vi "Ensaio_Jiga.vi"() -> ()   [LabVIEW 2025]
uses:
  Enum_Estados_Ensaio.ctl
  <vilib>/DAQmx/write.llb/DAQmx Write (Digital Bool 1Line 1Point).vi
  <vilib>/DAQmx/write.llb/DAQmx Write (Digital 1D Bool 1Chan 1Samp).vi
  <vilib>/Plasmionique/MB Master/MB_Master_Serial/MB_Master_Serial.lvclass
  C:/Program Files/National Instruments/LabVIEW 2025/vi.lib/Plasmionique/MB Master/MB_Master/MB_Master.lvclass
  <vilib>/DAQmx/create/channels.llb/DAQmx Create Channel (DO-Digital Output).vi
  <vilib>/DAQmx/miscellaneous.llb/DAQmx Fill In Error Info.vi
  <vilib>/Utility/file.llb/Write Delimited Spreadsheet (DBL).vi
  <vilib>/addons/control/pid/pid.llb/PID Gain Schedule (DBL).vi
  <vilib>/addons/control/pid/pid.llb/PID Advanced (DBL).vi
  <vilib>/Utility/file.llb/Write Delimited Spreadsheet (string).vi
  <instrlib>/Yokogawa PZ4000/Yokogawa PZ4000.lvlib
  <instrlib>/Yokogawa WT200 Series/Yokogawa WT200 Series.lvlib
  <vilib>/addons/control/pid/NI_PID_pid.lvlib
panel:
  out "Chart_velo":cluster{"V(A)":dbl, "V(B)":dbl}(graph)
  out "error out":errorcluster
  out "Registers":u16[](array[numeric])
  in  "Manual?":bool=TRUE
  in  "Medição contínua?":bool
  in  "Tempo de Integração":dbl=5.0
  in  "Realiza medição WT230":bool
  out "Tensão de Saída":dbl
  out "Corrente de Saída":dbl
  in  "Limite Tensao":dbl=24.0 min=0.0 max=36.0 step=0.5
  in  "Limite Corrente":dbl min=0.0 max=0.2 step=0.01
  in  "Para Freio":bool
  in  "Seta Carga":bool
  in  "Liga Fonte":bool
  in  "Iniciar Ensaio":bool
  in  "Finalizar Sessão":bool
  in  "ABORTAR":bool
  in  "?":T1(tab)
  out "Ensaio Rodando":bool
  in  "N_Resistores":string="1000"
  in  "Qtd. Braços Ativos":dbl min=0.0 max=7.0 step=1.0
  in  "Tempo de Pré-Carga (s)":dbl=90.0
  in  "Tempo de Acionamento do Motor (s)":dbl=14.0
  in  "Salvar Ensaio":path
  in  "VISA Resource":refnum<visa-resource-name>="COM3"
  in  "velocidade":u16
  in  "Serial Config":T2={"baud rate (bps)"=9600, "stop bits"=10, "parity"=2, "flow control"=0, "timeout"=2000, "retries"=3} {"stop bits" items=["1.0"=10, "1.5"=15, "2.0"=20]; "flow control" items=["None", "XON/XOFF", "RTS/CTS", "XON/XOFF & RTS/CTS", "DTR/DSR", "XON/XOFF & DTR/DSR"]; "parity" items=["None", "Odd", "Even", "Mark", "Space"]}
  in  "habilitar":u16=256
  out "Ganho atual do PI MI":T3={"proportional gain (Kc)"=100.0, "integral time (Ti, min)"=0.0, "derivative time (Td, min)"=0.0} {"derivative time (Td, min)" format="%.3f"; "integral time (Ti, min)" format="%.3f"; "proportional gain (Kc)" format="%.5f"}
  in  "SP_Power":i32
  out "Tempo Decorrido Acionamento Motor":dbl
  in  "Resistor 2 068":bool caption="4º Resistor 2 068"
  in  "Resistor 2 047":bool caption="3º Resistor 2 047"
  in  "Resistor 1  047":bool caption="2º Resistor 1  047"
  in  "Resistor 1 MOSFET":bool caption="1º Resistor 1 MOSFET"
  in  "PARAR WHILE":bool
  out "Estado Atual":T4
  out "V Cluster":cluster{"V(A)":dbl, "V(B)":dbl, "V(E)":dbl}
  out "I Cluster":cluster{"V(A)":dbl, "V(B)":dbl, "V(E)":dbl}
  out "P Cluster":T5
  out "PV_PowerControl":dbl
  in  "Ganhos PI do Gain Scheduling":T6(array[cluster])=[{"PID Parameters"={"Kc"=0.00026, "  Ti"=0.027, " Td"=0.0}, "Max PV"=490.0}, {"PID Parameters"={"Kc"=0.00027, "  Ti"=0.037, " Td"=0.0}, "Max PV"=690.0}, {"PID Parameters"={"Kc"=0.00019, "  Ti"=0.024, " Td"=0.0}, "Max PV"=900.0}] {"Max PV" format="%#.2f"; "PID Parameters"."Td" format="%#.3g"; "PID Parameters"."Ti" format="%#.3g"; "PID Parameters"."Kc" format="%#.5f"}
  in  "Ts Controle":dbl=0.1
  out "MV_MI":dbl=5.583364480052211
  out "Grafico_VelocidadeMotor":u16[](graph) caption="Velocidade do Motor"
  in  "Logfile_Watt":string="medsWatt"
  in  "Logfile_Freio":string="medsFreio"
  out "t":dbl
  in  "Logfile_ETMI":string="medsETMI"
  out "Corrente":dbl[][](graph)
  out "Tensão":dbl[][](graph)
  out "Graf_MV_MI":dbl(graph)
  out "Grafico_PowerControl":cluster{"PV_PowerControl":dbl, "SP_Power":i32}(graph)
  in  "Iniciar Acionamento":bool
  # "Aquisição WT230"
  # "CONTROLES DO ENSAIO"
  # "FREIO DE HISTERESE"
  # "Motor"
  # "Atenção: Antes de todo ensaio configurar o arquivo de saída para o padrão - Ensaio_{QtdBracos}bracos_RSE{ValorRSE}_SemCarga_{DataHora}.csv"
  # "Exemplo: 0Bracos_R1000_80W_2026-09-17_14_00.csv"
  # "BRAÇOS DE RESISTORES"
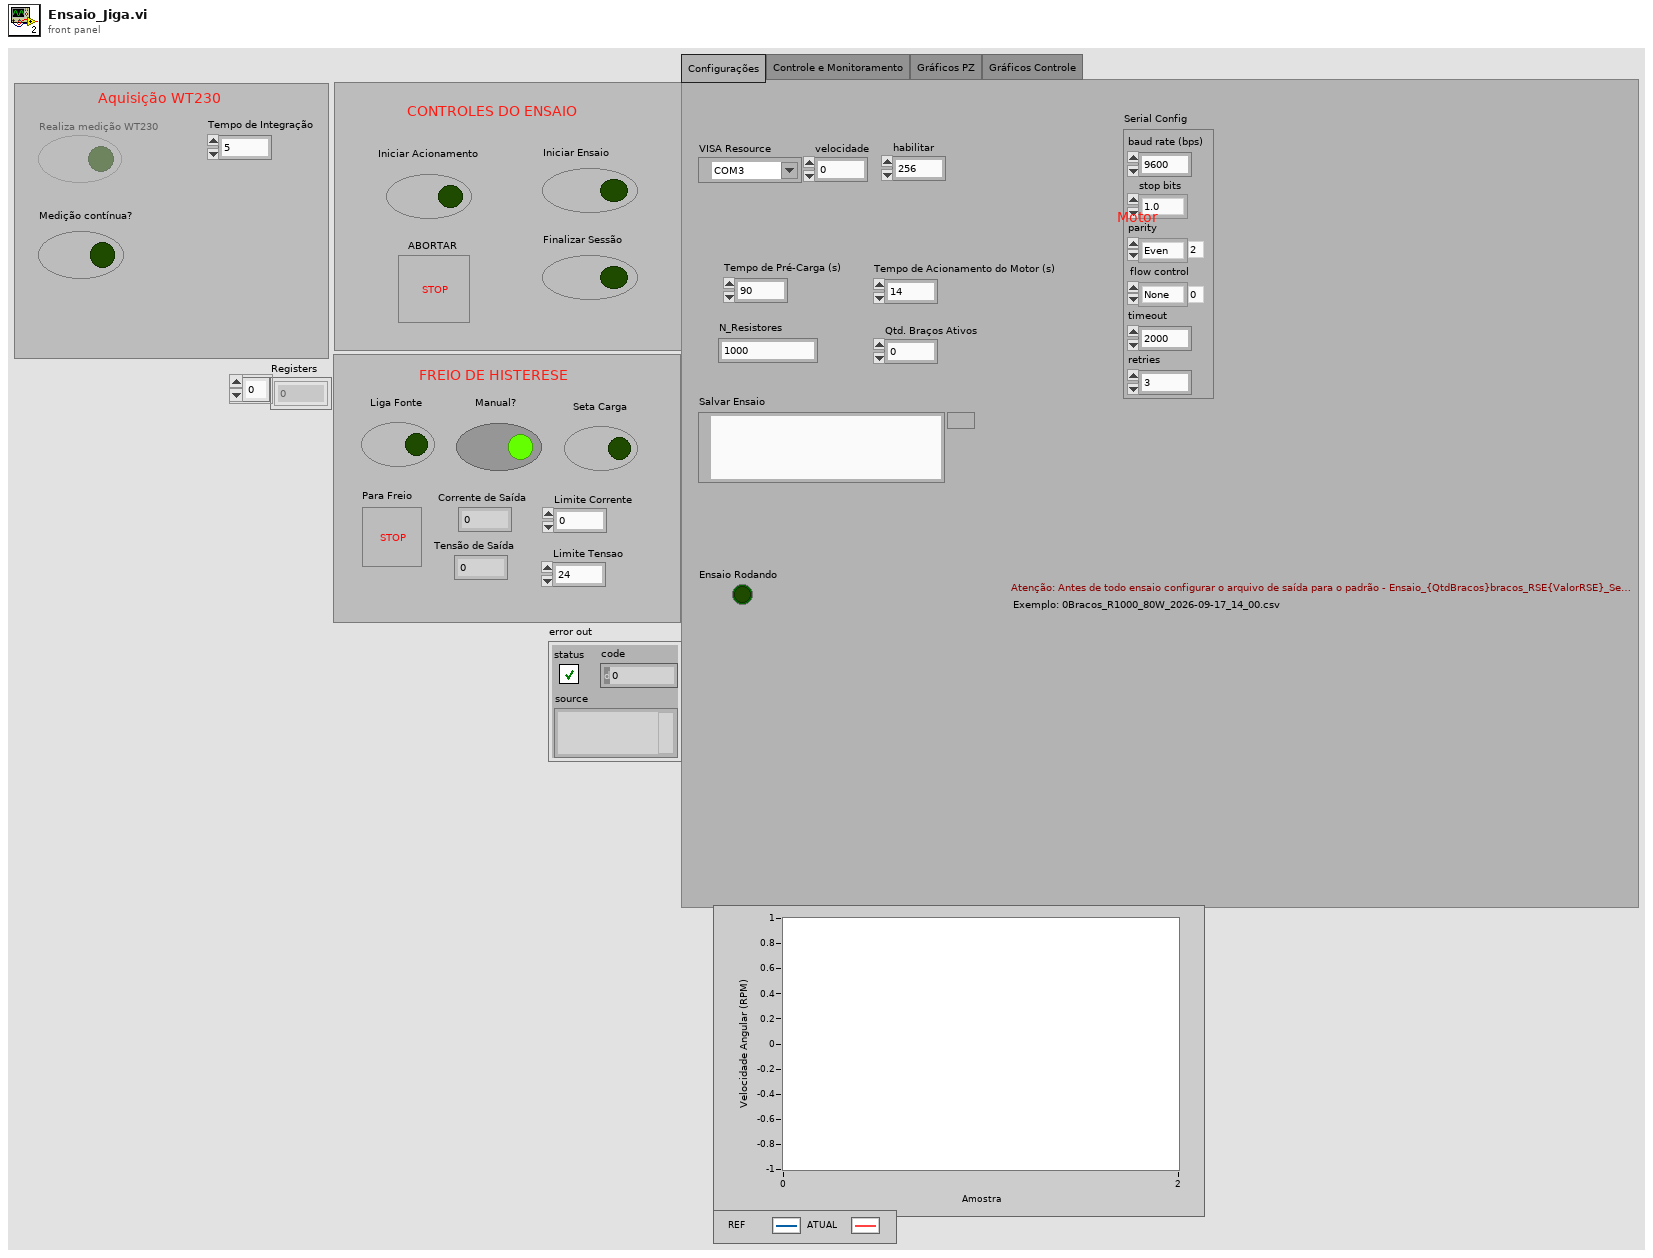
[diagram p1: front panel]
types:
  T1 = enum32{"Configurações", "Controle e Monitoramento", "Gráficos PZ", "Gráficos Controle"}
  T2 = cluster{"baud rate (bps)":u32, "stop bits":u16, "parity":u16, "flow control":u16, "timeout":u32, "retries":i32}
  T3 = cluster{"proportional gain (Kc)":dbl, "integral time (Ti, min)":dbl, "derivative time (Td, min)":dbl}
  T4 = typedef "Enum_Estados_Ensaio.ctl" = enum16{"Idle", "Pre_Carga", "Aguarda_PreCarga", "Ativa_Bracos", "Delay_PosBracos", "Desativa_PreCarga", "Aciona_Motor", "Aguarda_Motor", "Motor_Rodando", "Ensaio", "Para_Motor", "Emergencia\n"}
  T5 = cluster{"output":dbl, "output":dbl, "output":dbl, "PL(A)":dbl, "PL(B)":dbl, "PL(T)":dbl, "output":dbl, "PL(E)":dbl}
  T6 = cluster{"PID Parameters":cluster{"Kc":dbl, "  Ti":dbl, " Td":dbl}, "Max PV":dbl}[]
  T7 = enum8{"Enabled", "Disabled", "Disabled and Grayed Out"}
  T8 = cluster{"V(A)":dbl, "I(A)":dbl, "V(B)":dbl, "I(B)":dbl, "PC(A)":dbl, "PC(B)":dbl, "PC(T)":dbl, "PL(T)":dbl, "PL(B)":dbl, "PL(A)":dbl, "V(E)":dbl, "PL(E)":dbl, "PC(E)":dbl, "I(E)":dbl, "t":dbl}
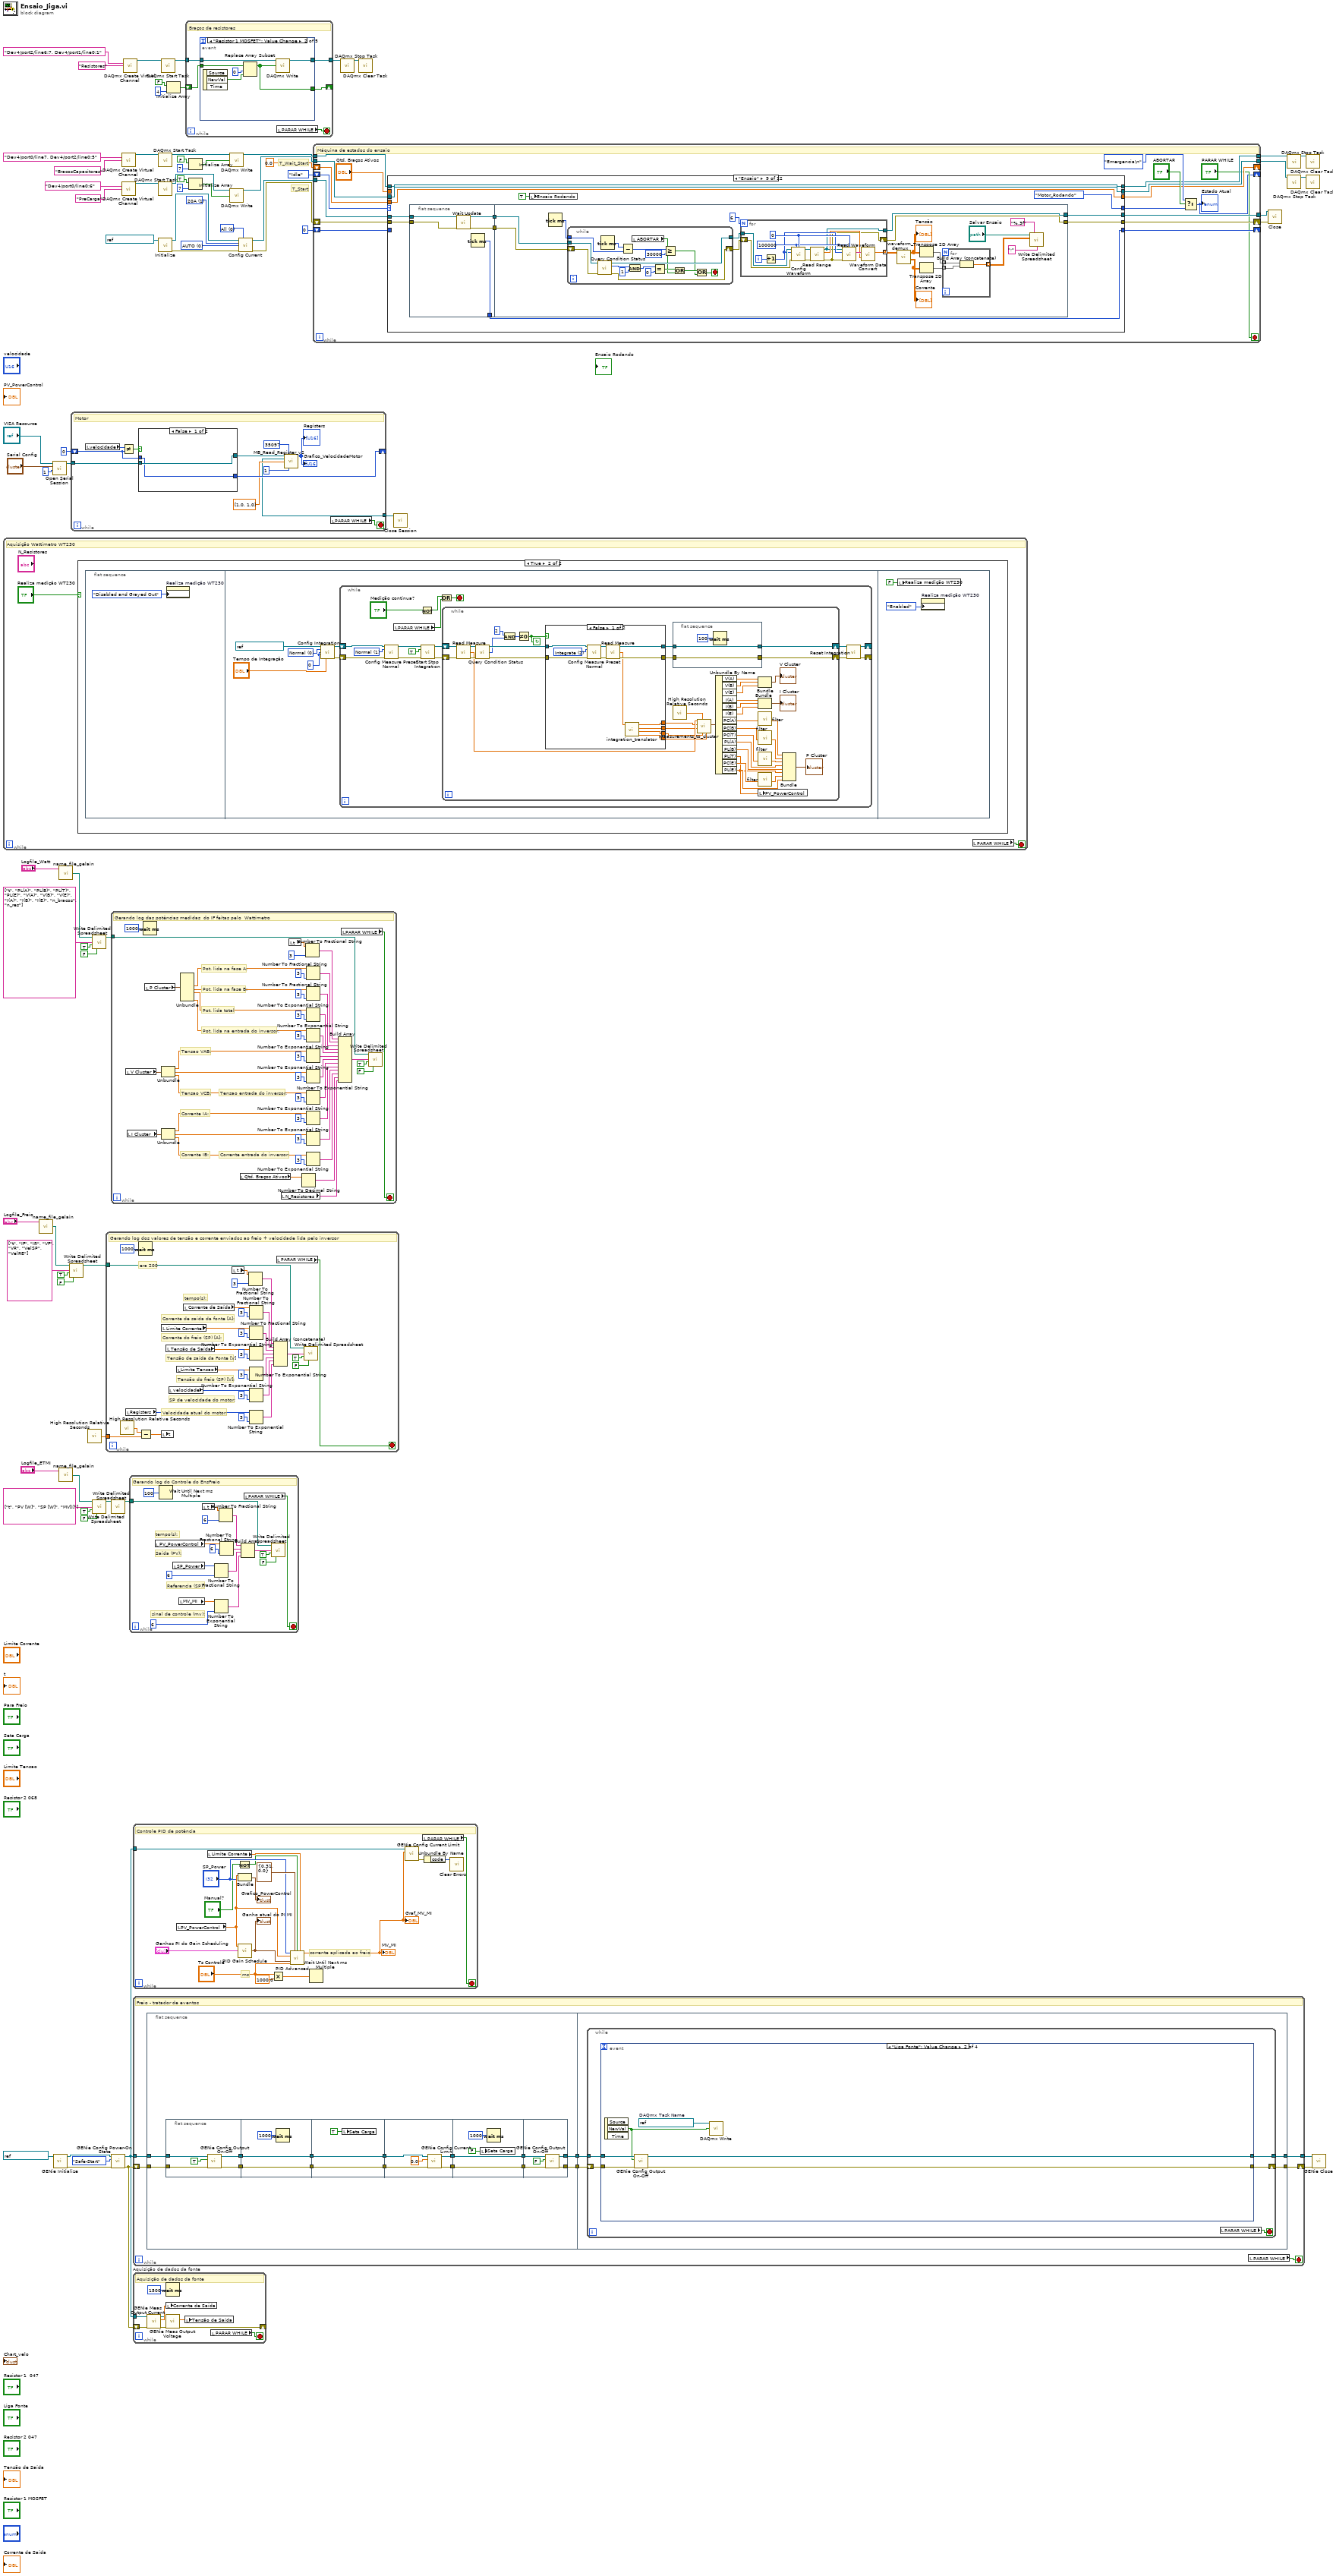
[diagram p0: block diagram]
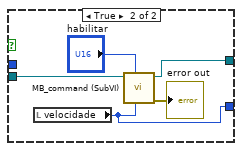
[diagram p2: hidden frame]
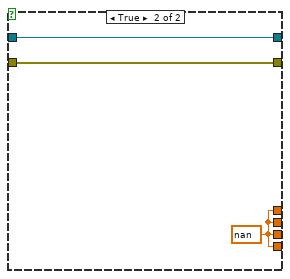
[diagram p4: hidden frame]
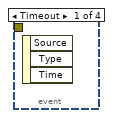
[diagram p5: hidden frame]
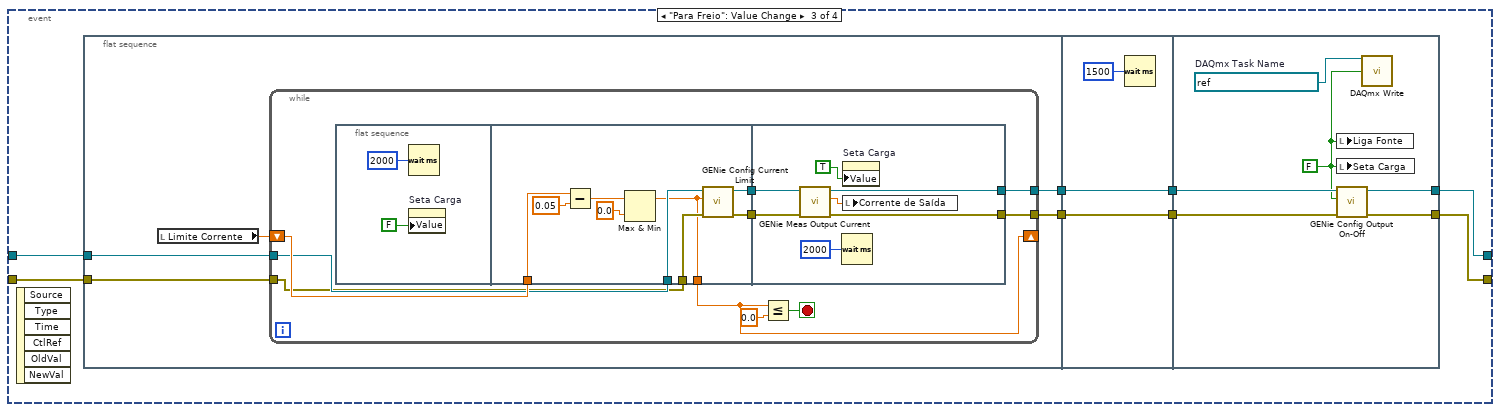
[diagram p6: hidden frame]
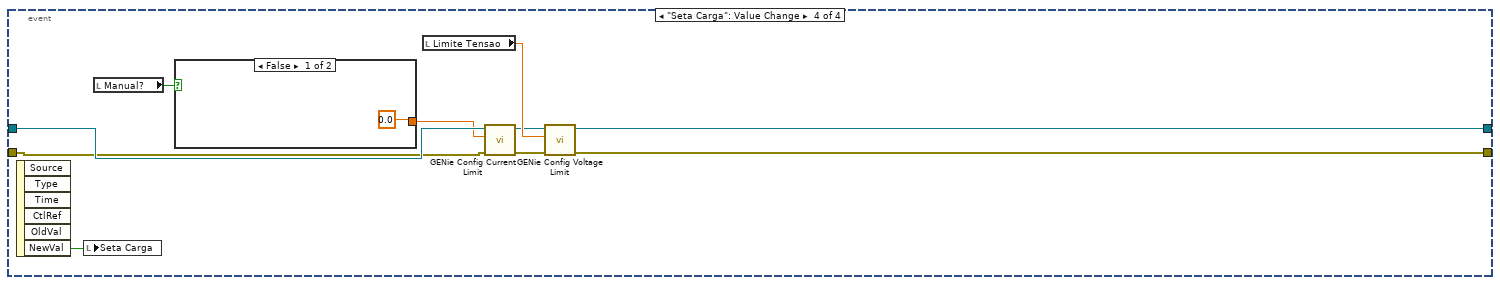
[diagram p7: hidden frame]
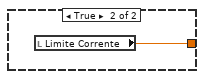
[diagram p8: hidden frame]
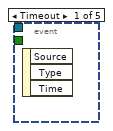
[diagram p9: hidden frame]
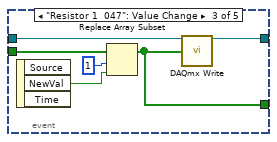
[diagram p10: hidden frame]
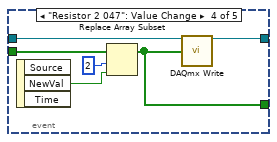
[diagram p11: hidden frame]
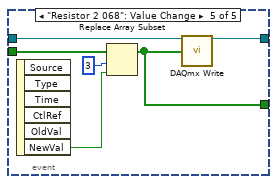
[diagram p12: hidden frame]
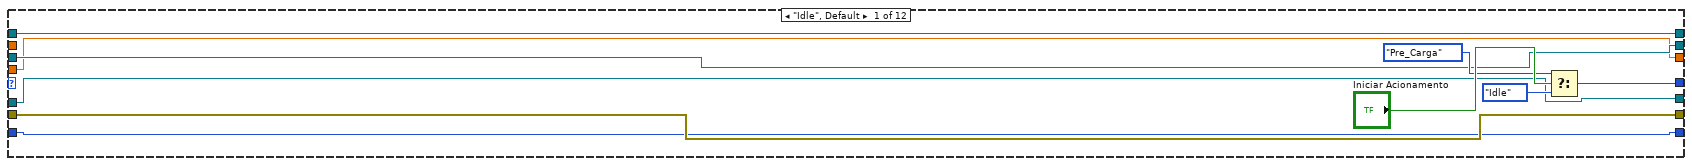
[diagram p13: hidden frame]
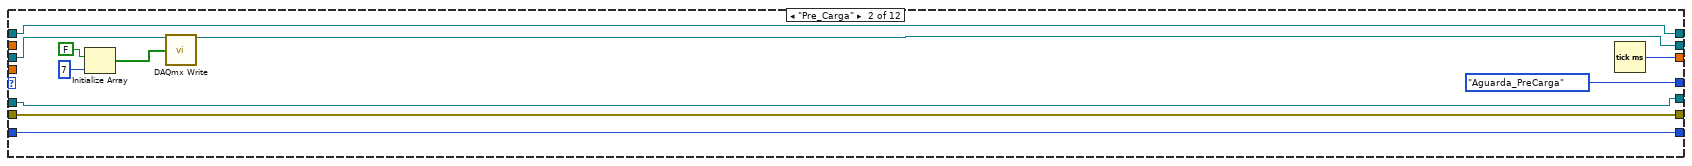
[diagram p14: hidden frame]
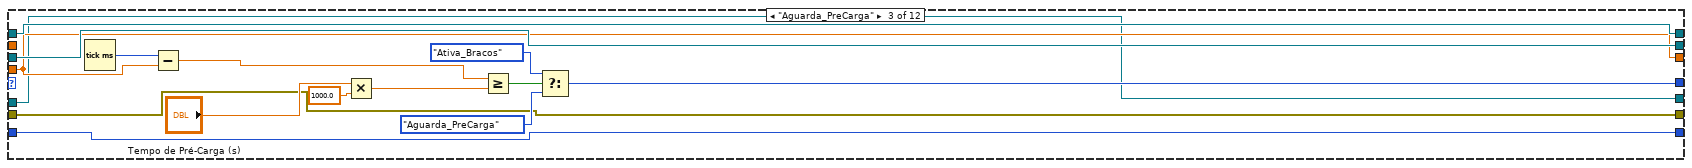
[diagram p15: hidden frame]
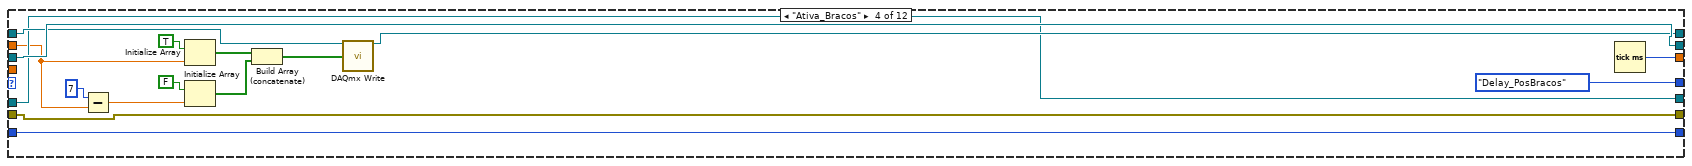
[diagram p16: hidden frame]
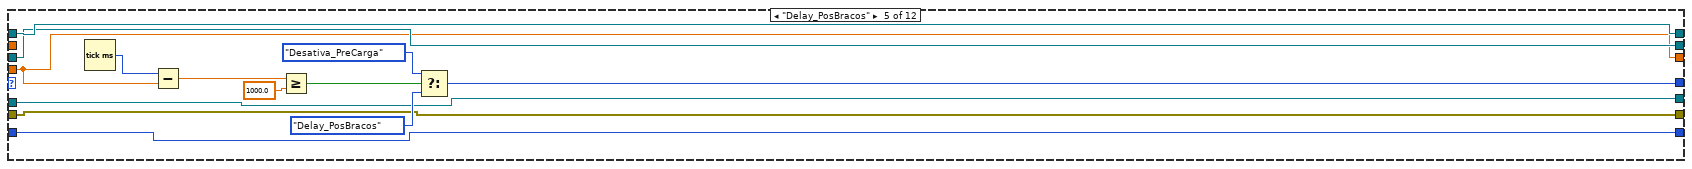
[diagram p17: hidden frame]
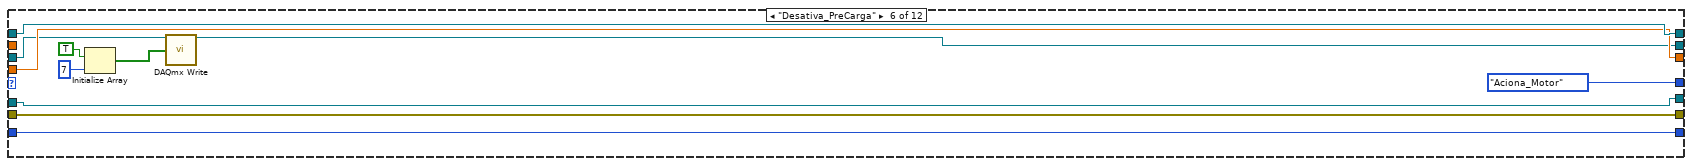
[diagram p18: hidden frame]
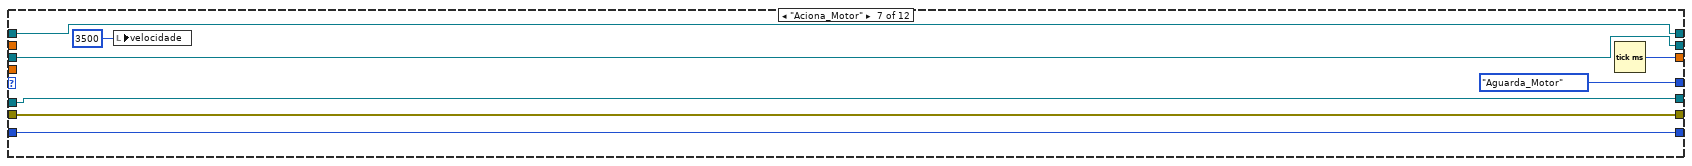
[diagram p19: hidden frame]
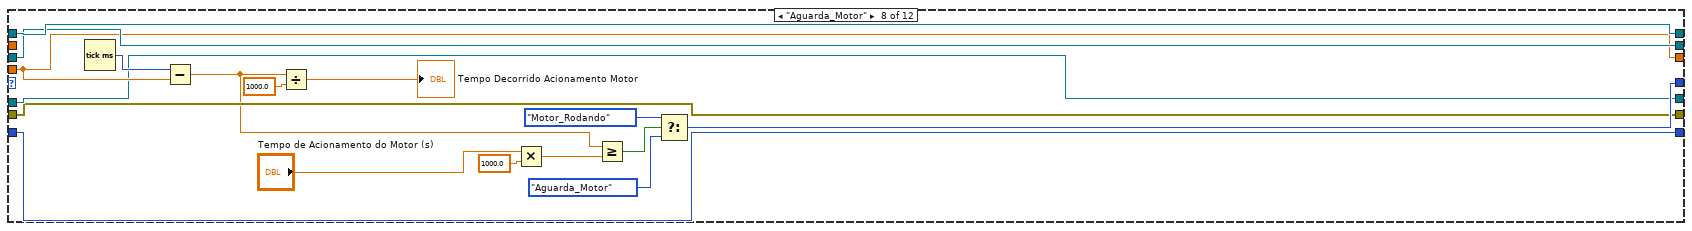
[diagram p20: hidden frame]
diagram:
  w45 = u16 0 items=["AUTO", "0.1", "0.2", "0.4", "1", "2", "4", "10", "20", "40", "100"] ("A Range (7:10)")
  w46 = u16 1 items=["5A", "20A", "Sensor"] ("A Terminal (0: 5A)")
  w47 = u16 0 items=["All", "Element 1", "Element 2", "Element 3", "Element 4"] ("Element (0: ALL)")
  # "T_Start"
  # "T_Wait_Start"
  n1 = while {
    stop <- w77 stop-if-true
    # "Aquisição Wattímetro WT230"
    n2 = case shown="True" "Realiza medição WT230" {
      frame False {
      }
      frame True {
        n3 = flat-sequence {
          frame #0 {
            n4 = property on="Realiza medição WT230" class="Bool (strict)"("DisabledEnum"=T7."Disabled and Grayed Out" ("Disabled")) -> ()  [unwired: 2 in, 2 out]
          }
          frame #1 {
            w83 = u32 0 ("Hour (0)")
            w84 = u16 0 items=["Normal", "Continuous"] ("Integ Mode (0: Normal)")
            n5 = call <instrlib>:"Config Integration.vi"("VISA resource name"=refnum<visa-resource-name> "GPIB0::8::INSTR", "Integ Mode (0: Normal)"=w84, "Hour (0)"=w83, "Minute (0)"=w83, "Second (0)"="Tempo de Integração") -> ("VISA resource name out"=w81:refnum<visa-resource-name>, "error out"=w80:errorcluster)  [unwired: 9 in]
            n6 = while {
              shift-right: [w87] -> _
              shift-left: w81 -> [w101]
              shift-right: [w86] -> _
              shift-left: w80 -> [w100]
              stop <- w92 stop-if-true
              w99 = u16 1 items=["Clear", "Normal", "Integrate"] ("Preset Pattern (0: Clear)")
              n7 = call <instrlib>:"Config Measure Preset Normal.vi"("VISA resource name"=w101, "Preset Pattern (0: Clear)"=w99, "error in (no error)"=w100) -> ("VISA resource name out"=w98:refnum<visa-resource-name>, "error out"=w97:errorcluster)  [unwired: 11 in]
              n8 = local read "PARAR WHILE"() -> (w93:bool)
              n9 = Not(x="Medição contínua?") -> (.not. x?=w94:bool)
              n10 = call <instrlib>:"Start Stop Integration.vi"("VISA resource name"=w98, "Start/Stop (F: Stop)"=TRUE, "error in (no error)"=w97) -> ("VISA resource name out"=w91:refnum<visa-resource-name>, "error out"=w90:errorcluster)  [unwired: 11 in]
              n11 = Or(x=w94, y=w93) -> (x .or. y?=w92:bool)
              n12 = while {
                shift-right: [w125] -> w89
                shift-left: w91 -> [w143]
                shift-right: [w124] -> w88
                shift-left: w90 -> [w142]
                stop <- w133 continue-if-true
                n13 = call <instrlib>:"Read Measure.vi"("VISA resource name"=w143, "error in (no error)"=w142) -> ("VISA resource name out"=w141:refnum<visa-resource-name>, "Measure Value"=w134:sgl[], "error out"=w140:errorcluster)  [unwired: 10 in, 1 out]
                n14 = call <instrlib>:"Query Condition Status.vi"("VISA resource name"=w141, "error in (no error)"=w140) -> ("VISA resource name out"=w139:refnum<visa-resource-name>, "Condition"=w137:u16, "error out"=w138:errorcluster)  [unwired: 11 in]
                n15 = And(x=u16 2, y=w137) -> (x .and. y?=w135:u16)
                n16 = Not Equal To 0?(x=w135) -> (x != 0?=w133:bool)
                n17 = case shown="False" w133 {
                  tunnel: w139 -> [w158 w161]
                  tunnel: w138 -> [w157 w160]
                  tunnel: [w153 w161] -> w126
                  tunnel: [w152 w160] -> w127
                  tunnel: [w150 w159] -> w132
                  tunnel: [w149 w159] -> w131
                  tunnel: [w148 w159] -> w130
                  tunnel: [w147 w159] -> w129
                  frame False {
                    w156 = u16 2 items=["Clear", "Normal", "Integrate"] ("Preset Pattern (0: Clear)")
                    n18 = call <instrlib>:"Config Measure Preset Normal.vi"("VISA resource name"=w158, "Preset Pattern (0: Clear)"=w156, "error in (no error)"=w157) -> ("VISA resource name out"=w155:refnum<visa-resource-name>, "error out"=w154:errorcluster)  [unwired: 11 in]
                    n19 = call <instrlib>:"Read Measure.vi"("VISA resource name"=w155, "error in (no error)"=w154) -> ("VISA resource name out"=w153:refnum<visa-resource-name>, "Measure Value"=w151:sgl[], "error out"=w152:errorcluster)  [unwired: 10 in, 1 out]
                    n20 = call "integration_translator.vi"("Valores integração"=w151) -> ("PI(E)"=w147:sgl, "PI(T)"=w148:sgl, "PI(B)"=w149:sgl, "PI(A)"=w150:sgl)  [unwired: 7 in]
                  }
                  frame True {
                    w159 = sgl nan ("PI(B)")
                  }
                }
                n21 = flat-sequence {
                  tunnel: [w145] -> w124
                  tunnel: w127 -> [w145]
                  tunnel: w126 -> [w144]
                  tunnel: [w144] -> w125
                  frame #0 {
                    n22 = Wait (ms)(milliseconds to wait=u32 100) -> ()  [unwired: 1 out]
                  }
                }
                n23 = call <vilib>:"High Resolution Relative Seconds.vi"() -> ("relative seconds"=w128:dbl)
                n24 = call "measurements_to_cluster.vi"("PI(E)"=w129, "PI(T)"=w130, "relative seconds"=w128, "PI(B)"=w131, "PI(A)"=w132, "Measure Value"=w134) -> ("watt cluster"=w123:T8)  [unwired: 4 in, 1 out]
                n25 = Unbundle By Name(w123) -> ("V(A)"=w118:dbl, "V(B)"=w117:dbl, "V(E)"=w116:dbl, "I(A)"=w115:dbl, "I(B)"=w114:dbl, "I(E)"=w113:dbl, "PC(A)"=w122:dbl, "PC(B)"=w121:dbl, "PC(T)"=w120:dbl, "PL(A)"=w109:dbl, "PL(B)"=w108:dbl, "PL(T)"=w105:dbl, "PC(E)"=w119:dbl, "PL(E)"=w106:dbl)
                n26 = Bundle("V(A)"=w118, "V(B)"=w117, "V(E)"=w116) -> (→"V Cluster":cluster{"V(A)":dbl, "V(B)":dbl, "V(E)":dbl})  [unwired: 1 in]
                n27 = Bundle("I(A)"=w115, "I(B)"=w114, "I(E)"=w113) -> (→"I Cluster":cluster{"I(A)":dbl, "I(B)":dbl, "I(E)":dbl})  [unwired: 1 in]
                n28 = call "filter.vi"("input"=w122) -> ("output"=w112:dbl)  [unwired: 10 in]
                n29 = call "filter.vi"("input"=w121) -> ("output"=w111:dbl)  [unwired: 10 in]
                n30 = call "filter.vi"("input"=w120) -> ("output"=w110:dbl)  [unwired: 10 in]
                n31 = call "filter.vi"("input"=w119) -> ("output"=w107:dbl)  [unwired: 10 in]
                n32 = local write "PV_PowerControl"(w105) -> ()
                n33 = Bundle("output"=w112, "output"=w111, "output"=w110, "PL(A)"=w109, "PL(B)"=w108, "PL(T)"=w105, "output"=w107, "PL(E)"=w106) -> (→"P Cluster":T5)  [unwired: 1 in]
              }
              n34 = call <instrlib>:"Reset Integration.vi"("VISA resource name"=w89, "error in (no error)"=w88) -> ("VISA resource name out"=w87:refnum<visa-resource-name>, "error out"=w86:errorcluster)  [unwired: 12 in]
            }
          }
          frame #2 {
            n35 = local write "Realiza medição WT230"(FALSE ("Realiza medição WT230")) -> ()
            n36 = property on="Realiza medição WT230" class="Bool (strict)"("DisabledEnum"=T7."Enabled" ("Disabled")) -> ()  [unwired: 2 in, 2 out]
          }
        }
      }
    }
    n37 = local read "PARAR WHILE"() -> (w77:bool)
  }
  n38 = call "name_file_gelain.vi"("Identifier"="Logfile_Freio") -> ("appended path"=w6:path)  [unwired: 2 in]
  n39 = call <vilib>:"Open Serial Session.vi"("Slave ID"=u8 1, "Serial Config"="Serial Config", "VISA Resource"="VISA Resource") -> ("MB_Serial session"=w23:refnum<class "MB_Master_Serial.lvclass">)  [unwired: 7 in, 1 out]
  n40 = call <instrlib>:"GENie Initialize.vi"("VISA name"=refnum<visa-resource-name> "GPIB::6::INSTR") -> ("error out"=w30:errorcluster, "VISA out"=w34:refnum<visa-resource-name>)  [unwired: 9 in]
  n41 = call "name_file_gelain.vi"("Identifier"="Logfile_Watt") -> ("appended path"=w2:path)  [unwired: 2 in]
  n42 = call "name_file_gelain.vi"("Identifier"="Logfile_ETMI") -> ("appended path"=w4:path)  [unwired: 2 in]
  n43 = call-poly <vilib>:"Write Delimited Spreadsheet.vi"("file path (dialog if empty)"=w6, "1D data"=string[] ["t", "IF", "IR", "VF", "VR", "VelSP", "VelRE"], "append to file? (new file:F)"=TRUE, "transpose? (no:F)"=FALSE) -> ("new file path (Not A Path if cancelled)"=w14:path)  [unwired: 10 in, 1 out]
  n44 = while {
    tunnel: w23 -> [w172]
    shift-right: [w171] -> _
    shift-left: 0 -> [w170]
    tunnel: [w165] -> w21
    stop <- w175 stop-if-true
    # "Motor"
    n45 = local read "velocidade"() -> (w174:u16)
    n46 = Not Equal?(x=w174, y=w170) -> (x != y?=w173:bool)
    n47 = case shown="False" w173 {
      tunnel: w172 -> [w177 w180]
      tunnel: [w177 w179] -> w166
      tunnel: [w176 w178] -> w171
      tunnel: w170 -> [w176 _]
      frame False {
      }
      frame True {
        n48 = local read "velocidade"() -> (w178:u16)
        n49 = call "MB_command (SubVI).vi"("velocidade"=w178, "habilitar"="habilitar", "MB session in"=w180) -> ("error out"=→"error out":errorcluster, "MB session out"=w179:refnum<class "MB_Master_Serial.lvclass">)  [unwired: 7 in]
      }
    }
    n50 = call "MB_Read_Register_v2.vi"("MB session in"=w166, "starting address"=u16 35097, "ganho"=dbl[] [1.0, 1.0], "quantity"=u16 1) -> ("Registers"=→"Registers" →"Grafico_VelocidadeMotor":u16[], "MB session out"=w165:refnum<class "MB_Master_Serial.lvclass">)  [unwired: 9 in, 1 out]
    n51 = local read "PARAR WHILE"() -> (w175:bool)
  }
  n52 = call <vilib>:"High Resolution Relative Seconds.vi"() -> ("relative seconds"=w13:dbl)
  n53 = call-poly <vilib>:"Write Delimited Spreadsheet.vi"("file path (dialog if empty)"=w2, "1D data"=string[] ["t", "PL(A)", "PL(B)", "PL(T)", "PL(E)", "V(A)", "V(B)", "V(E)", "I(A)", "I(B)", "I(E)", "n_bracos", "n_res"] ("appended array"), "append to file? (new file:F)"=TRUE, "transpose? (no:F)"=FALSE) -> ("new file path (Not A Path if cancelled)"=w17:path)  [unwired: 10 in, 1 out]
  n54 = call-poly <vilib>:"Write Delimited Spreadsheet.vi"("file path (dialog if empty)"=w4, "1D data"=string[] ["t", "PV [W]", "SP [W]", "MV[I]"] ("appended array"), "append to file? (new file:F)"=TRUE, "transpose? (no:F)"=FALSE) -> ("new file path (Not A Path if cancelled)"=w8:path)  [unwired: 10 in, 1 out]
  n55 = while {
    tunnel: w14 -> [w210]
    tunnel: w13 -> [w195]
    stop <- w186 stop-if-true
    # "Velocidade atual do motor:"
    # "SP de velocidade do motor:"
    # "era 200"
    # "Tensão do freio (SP) [V]:"
    # "tempo(s):"
    # "Corrente de saída da fonte [A]:"
    # "Corrente do freio (SP) [A]:"
    # "Tensão de saída da Fonte [V]"
    # "Gerando log dos valores de tensão e corrente enviados ao freio + velocidade lida pelo inversor"
    n56 = call <vilib>:"High Resolution Relative Seconds.vi"() -> ("relative seconds"=w196:dbl)
    n57 = local read "Registers"() -> (w187:u16[])
    n58 = Wait (ms)(milliseconds to wait=u32 1000) -> ()  [unwired: 1 out]
    n59 = Subtract(x=w196, y=w195) -> (x-y=w185:dbl)
    n60 = local read "Limite Corrente"() -> (w190:dbl)
    n61 = local write "t"(w185) -> ()
    n62 = local read "Tensão de Saída"() -> (w183:dbl)
    n63 = local read "velocidade"() -> (w188:u16)
    n64 = local read "Limite Tensao"() -> (w189:dbl)
    n65 = local read "Corrente de Saída"() -> (w184:dbl)
    n66 = local read "t"() -> (w205:dbl)
    n67 = Number To Fractional String(number=w205, precision (6)=i16 3) -> (F-format string=w204:string)  [unwired: 2 in]
    n68 = Number To Fractional String(number=w184, precision (6)=i16 3) -> (F-format string=w203:string)  [unwired: 2 in]
    n69 = Number To Fractional String(number=w190, precision (6)=i16 3) -> (F-format string=w200:string)  [unwired: 2 in]
    n70 = Number To Exponential String(number=w183, precision (6)=i16 3) -> (E-format string=w208:string)  [unwired: 2 in]
    n71 = Number To Exponential String(number=w189, precision (6)=i16 3) -> (E-format string=w197:string)  [unwired: 2 in]
    n72 = Number To Exponential String(number=w188, precision (6)=i16 3) -> (E-format string=w193:string)  [unwired: 2 in]
    n73 = Number To Exponential String(number=w187, precision (6)=i16 3) -> (E-format string=w191:string[])  [unwired: 2 in]
    n74 = Build Array (concatenate)(w204, w203, w200, w208, w197, w193, w191) -> (w201:string[])
    n75 = local read "PARAR WHILE"() -> (w186:bool)
    n76 = call-poly <vilib>:"Write Delimited Spreadsheet.vi"("file path (dialog if empty)"=w210, "1D data"=w201, "append to file? (new file:F)"=TRUE, "transpose? (no:F)"=FALSE) -> ()  [unwired: 10 in, 2 out]
  }
  n77 = while {
    tunnel: w17 -> [w255]
    stop <- w219 stop-if-true
    # "Corrente IB:"
    # "Corrente entrada do inversor:"
    # "Corrente IA:"
    # "Tensao entrada do inversor:"
    # "Tensao VCB:"
    # "Tensao VAB:"
    # "Pot. lida na entrada do inversor:"
    # "Pot. lida total"
    # "Pot. lida na fase A:"
    # "Pot. lida na fase B:"
    # "Gerando log das potências medidas  do IF feitas pelo  Wattímetro"
    n78 = local read "V Cluster"() -> (w220:cluster{"V(A)":dbl, "V(B)":dbl, "V(E)":dbl})
    n79 = local read "I Cluster"() -> (w221:cluster{"V(A)":dbl, "V(B)":dbl, "V(E)":dbl})
    n80 = Wait (ms)(milliseconds to wait=u32 1000) -> ()  [unwired: 1 out]
    n81 = local read "P Cluster"() -> (w222:T5)
    n82 = Unbundle(w220) -> ("V(A)"=w229:dbl, "V(B)"=w233:dbl, "V(E)"=w223:dbl)
    n83 = Unbundle(w221) -> ("V(A)"=w232:dbl, "V(B)"=w231:dbl, "V(E)"=w230:dbl)
    n84 = Unbundle(w222) -> ("PL(A)"=w242:dbl, "PL(B)"=w234:dbl, "PL(T)"=w241:dbl, "PL(E)"=w240:dbl)  [unwired: 4 out]
    n85 = local read "Qtd. Braços Ativos"() -> (w215:dbl)
    n86 = local read "N_Resistores"() -> (w213:string)
    n87 = local read "t"() -> (w216:dbl)
    n88 = Number To Decimal String(number=w215) -> (decimal integer string=w214:string)  [unwired: 1 in]
    n89 = Number To Fractional String(number=w216, precision (6)=i16 3) -> (F-format string=w217:string)  [unwired: 2 in]
    n90 = Number To Fractional String(number=w242, precision (6)=i16 3) -> (F-format string=w251:string)  [unwired: 2 in]
    n91 = Number To Fractional String(number=w234, precision (6)=i16 3) -> (F-format string=w248:string)  [unwired: 2 in]
    n92 = Number To Exponential String(number=w241, precision (6)=i16 3) -> (E-format string=w253:string)  [unwired: 2 in]
    n93 = Number To Exponential String(number=w240, precision (6)=i16 3) -> (E-format string=w246:string)  [unwired: 2 in]
    n94 = Number To Exponential String(number=w229, precision (6)=i16 3) -> (E-format string=w243:string)  [unwired: 2 in]
    n95 = Number To Exponential String(number=w233, precision (6)=i16 3) -> (E-format string=w228:string)  [unwired: 2 in]
    n96 = Number To Exponential String(number=w223, precision (6)=i16 3) -> (E-format string=w227:string)  [unwired: 2 in]
    n97 = Number To Exponential String(number=w232, precision (6)=i16 3) -> (E-format string=w226:string)  [unwired: 2 in]
    n98 = Number To Exponential String(number=w231, precision (6)=i16 3) -> (E-format string=w225:string)  [unwired: 2 in]
    n99 = Number To Exponential String(number=w230, precision (6)=i16 3) -> (E-format string=w224:string)  [unwired: 2 in]
    n100 = Build Array(w217, w251, w248, w253, w246, w243, w228, w227, w226, w225, w224, w214, w213) -> (w249:string[])
    n101 = local read "PARAR WHILE"() -> (w219:bool)
    n102 = call-poly <vilib>:"Write Delimited Spreadsheet.vi"("file path (dialog if empty)"=w255, "1D data"=w249, "append to file? (new file:F)"=TRUE, "transpose? (no:F)"=FALSE) -> ()  [unwired: 10 in, 2 out]
  }
  n103 = call-poly <vilib>:"Write Delimited Spreadsheet.vi"("file path (dialog if empty)"=w8) -> ("new file path (Not A Path if cancelled)"=w9:path)  [unwired: 13 in, 1 out]
  n104 = call <instrlib>:"GENie Config Power-On State.vi"("error"=w30, "Power-On"=enum16{"Safe-Start", "Auto-Start"}."Safe-Start", "VISA"=w34) -> ("error out"=w29:errorcluster, "VISA out"=w27:refnum<visa-resource-name>)  [unwired: 7 in]
  n105 = call-poly <vilib>:"DAQmx Create Virtual Channel.vi"("lines"=tag "Dev4/port0/line7, Dev4/port2/line0:5", "name to assign"="BracosCapacitores") -> ("task out"=w70:refnum<k21>)  [unwired: 12 in, 1 out]
  n106 = call-poly <vilib>:"DAQmx Create Virtual Channel.vi"("lines"=tag "Dev4/port0/line0:6", "name to assign"="PreCarga") -> ("task out"=w73:refnum<k21>)  [unwired: 12 in, 1 out]
  n107 = call-poly <vilib>:"DAQmx Create Virtual Channel.vi"("lines"=tag "Dev4/port2/line6:7, Dev4/port1/line0:1", "name to assign"="Resistores") -> ("task out"=w58:refnum<k21>)  [unwired: 12 in, 1 out]
  n108 = while {
    tunnel: w9 -> [w273]
    stop <- w258 stop-if-true
    # "tempo(s):"
    # "Saída (PV):"
    # "Referencia (SP):"
    # "sinal de controle (mv):"
    # "Gerando log do Controle do EnsFreio"
    n109 = local read "PV_PowerControl"() -> (w260:dbl)
    n110 = Wait Until Next ms Multiple(millisecond multiple=u32 100 ("milliseconds to wait")) -> ()  [unwired: 1 out]
    n111 = local read "SP_Power"() -> (w259:i32)
    n112 = local read "MV_MI"() -> (w261:dbl)
    n113 = local read "t"() -> (w262:dbl)
    n114 = Number To Fractional String(number=w259, precision (6)=i16 6) -> (F-format string=w264:string)  [unwired: 2 in]
    n115 = Number To Exponential String(number=w261, precision (6)=i16 6) -> (E-format string=w271:string)  [unwired: 2 in]
    n116 = Number To Fractional String(number=w262, precision (6)=i16 6) -> (F-format string=w268:string)  [unwired: 2 in]
    n117 = Number To Fractional String(number=w260, precision (6)=i16 6) -> (F-format string=w267:string)  [unwired: 2 in]
    n118 = Build Array(w268, w267, w264, w271) -> (w265:string[])
    n119 = local read "PARAR WHILE"() -> (w258:bool)
    n120 = call-poly <vilib>:"Write Delimited Spreadsheet.vi"("file path (dialog if empty)"=w273, "1D data"=w265, "append to file? (new file:F)"=TRUE, "transpose? (no:F)"=FALSE) -> ()  [unwired: 10 in, 2 out]
  }
  n121 = while {
    tunnel: w27 -> [w276]
    stop <- w292 stop-if-true
    # "corrente aplicada ao freio"
    # "ms"
    # "Controle PID de potência"
    n122 = local read "PV_PowerControl"() -> (w280:dbl)
    n123 = local read "Limite Corrente"() -> (w291:dbl)
    n124 = Not(x="Manual?") -> (.not. x?=w278:bool)
    n125 = Bundle("PV_PowerControl"=w280, "SP_Power"="SP_Power") -> (→"Grafico_PowerControl":cluster{"PV_PowerControl":dbl, "SP_Power":i32})  [unwired: 1 in]
    n126 = call-poly <vilib>:"PID Gain Schedule.vi"("PID gain schedule"="Ganhos PI do Gain Scheduling", "gain scheduling value"=w280) -> ("PID gains out"=w288:T3)  [unwired: 2 in, 1 out]
    "Ganho atual do PI MI" <- w288
    n127 = Multiply(x="Ts Controle", y=1000.0) -> (x*y=w287:dbl)
    n128 = call-poly <vilib>:"PID Advanced.vi"("setpoint"="SP_Power", "output range"=cluster{"output high":dbl, "output low":dbl} {"output high"=0.31, "output low"=0.0}, "auto? (T)"=w278, "manual control"=w291, "process variable"=w280, "PID gains"=w288, "dt (s)"="Ts Controle") -> ("output"=w282:dbl)  [unwired: 7 in, 1 out]
    "MV_MI" <- w282
    "Graf_MV_MI" <- w282
    n129 = Wait Until Next ms Multiple(millisecond multiple=w287) -> ()  [unwired: 1 out]
    n130 = call <instrlib>:"GENie Config Current Limit.vi"("Current Limit"=w282, "VISA"=w276) -> ("error out"=w283:errorcluster)  [unwired: 8 in, 1 out]
    n131 = local read "PARAR WHILE"() -> (w292:bool)
    n132 = Unbundle By Name(w283) -> ("code"=w284:i32)
    n133 = call <vilib>:"Clear Errors.vi"("specific error code to clear (0: all)"=w284) -> ()  [unwired: 5 in, 2 out]
  }
  n134 = while {
    shift-right: [w294] -> w28
    shift-left: w29 -> [w298]
    tunnel: w27 -> [w299]
    tunnel: [w293] -> w31
    stop <- w295 stop-if-true
    # "Freio - tratador de eventos"
    n135 = flat-sequence {
      tunnel: w299 -> [w303]
      tunnel: w298 -> [w302]
      tunnel: [w301] -> w297
      tunnel: [w300] -> w296
      tunnel: w297 -> [w342]
      tunnel: w296 -> [w341]
      tunnel: [w340] -> w294
      tunnel: [w339] -> w293
      frame #0 {
        n136 = flat-sequence {
          tunnel: w303 -> [w318]
          tunnel: w302 -> [w317]
          tunnel: [w315] -> w313
          tunnel: [w314] -> w312
          tunnel: w313 -> [w320]
          tunnel: w312 -> [w319]
          tunnel: [w320] -> w311
          tunnel: [w319] -> w310
          tunnel: w311 -> [w323]
          tunnel: w310 -> [w322]
          tunnel: [w323] -> w309
          tunnel: [w322] -> w308
          tunnel: w309 -> [w328]
          tunnel: w308 -> [w327]
          tunnel: [w326] -> w307
          tunnel: [w325] -> w306
          tunnel: w307 -> [w331]
          tunnel: w306 -> [w330]
          tunnel: [w331] -> w305
          tunnel: [w330] -> w304
          tunnel: w305 -> [w337]
          tunnel: w304 -> [w336]
          tunnel: [w335] -> w301
          tunnel: [w334] -> w300
          frame #0 {
            n137 = call <instrlib>:"GENie Config Output On-Off.vi"("error"=w317, "Output ON"=TRUE, "VISA"=w318) -> ("error out"=w314:errorcluster, "VISA out"=w315:refnum<visa-resource-name>)  [unwired: 7 in]
          }
          frame #1 {
            n138 = Wait (ms)(milliseconds to wait=u32 1000) -> ()  [unwired: 1 out]
          }
          frame #2 {
            n139 = local write "Seta Carga"(TRUE ("Seta Carga")) -> ()
          }
          frame #3 {
            n140 = call <instrlib>:"GENie Config Current Limit.vi"("error"=w327, "Current Limit"=0.0, "VISA"=w328) -> ("error out"=w325:errorcluster, "VISA out"=w326:refnum<visa-resource-name>)  [unwired: 7 in]
          }
          frame #4 {
            n141 = local write "Seta Carga"(FALSE ("Seta Carga")) -> ()
            n142 = Wait (ms)(milliseconds to wait=u32 1000) -> ()  [unwired: 1 out]
          }
          frame #5 {
            n143 = call <instrlib>:"GENie Config Output On-Off.vi"("error"=w336, "Output ON"=FALSE, "VISA"=w337) -> ("error out"=w334:errorcluster, "VISA out"=w335:refnum<visa-resource-name>)  [unwired: 7 in]
          }
        }
      }
      frame #1 {
        n144 = while {
          tunnel: w342 -> [w347]
          shift-right: [w344] -> w340
          shift-left: w341 -> [w346]
          tunnel: [w343] -> w339
          stop <- w345 stop-if-true
          n145 = event shown="[1] \"Liga Fonte\": Value Change" {
            selector: _ -> [_ _ _ _]
            dyn-events: _ -> [_ _ _ _]
            timeout: _ -> [_ _ _ _]
            tunnel: w347 -> [_ w353 w361 w412]
            tunnel: w346 -> [_ w352 w360 w411]
            tunnel: [_ w349 w355 w407] -> w344
            tunnel: [_ w348 w354 w406] -> w343
            event Timeout {
              n146 = event-data() -> ()  [unwired: 1 in, 3 out]
            }
            event "Liga Fonte": Value Change {
              w351 = refnum<k21> "resfriamento_freio"  # DAQmx Task Name
              n147 = event-data() -> ("NewVal"=w350:bool)  [unwired: 1 in, 2 out]
              n148 = call <instrlib>:"GENie Config Output On-Off.vi"("error"=w352, "Output ON"=w350, "VISA"=w353) -> ("error out"=w349:errorcluster, "VISA out"=w348:refnum<visa-resource-name>)  [unwired: 7 in]
              n149 = call-poly <vilib>:"DAQmx Write.vi"("task/channels in"=w351, "data"=w350) -> ()  [unwired: 11 in, 3 out]
            }
            event "Para Freio": Value Change {
              n150 = event-data() -> ()  [unwired: 1 in, 6 out]
              n151 = flat-sequence {
                tunnel: w361 -> [w365]
                tunnel: w360 -> [w364]
                tunnel: [w363] -> w358
                tunnel: [w362] -> w356
                tunnel: [w396] -> w359
                tunnel: w358 -> [w396]
                tunnel: [w395] -> w357
                tunnel: w356 -> [w395]
                tunnel: w359 -> [w402]
                tunnel: w357 -> [w401]
                tunnel: [w399] -> w355
                tunnel: [w398] -> w354
                frame #0 {
                  n152 = local read "Limite Corrente"() -> (w366:dbl)
                  n153 = while {
                    shift-right: [w369] -> _
                    shift-left: w366 -> [w376]
                    tunnel: w365 -> [w375]
                    tunnel: w364 -> [w374]
                    tunnel: [w368] -> w363
                    tunnel: [w367] -> w362
                    stop <- w373 stop-if-true
                    n154 = flat-sequence {
                      tunnel: w376 -> [w387]
                      tunnel: w375 -> [w385]
                      tunnel: w374 -> [w384]
                      tunnel: [w379] -> w369
                      tunnel: [w383] -> w371
                      tunnel: [w382] -> w370
                      tunnel: w371 -> [w393]
                      tunnel: w370 -> [w392]
                      tunnel: [w390] -> w368
                      tunnel: [w389] -> w367
                      frame #0 {
                        n155 = Wait (ms)(milliseconds to wait=u32 2000) -> ()  [unwired: 1 out]
                        n156 = property on="Seta Carga" class="Bool (strict)"("Value"=FALSE ("Seta Carga")) -> ()  [unwired: 2 in, 2 out]
                      }
                      frame #1 {
                        n157 = Subtract(x=w387, y=0.05) -> (x-y=w381:dbl)
                        n158 = Max & Min(x=w381, y=0.0) -> (max(x,y)=w379:dbl)  [unwired: 1 out]
                        n159 = call <instrlib>:"GENie Config Current Limit.vi"("error"=w384, "Current Limit"=w379, "VISA"=w385) -> ("error out"=w382:errorcluster, "VISA out"=w383:refnum<visa-resource-name>)  [unwired: 7 in]
                      }
                      frame #2 {
                        n160 = call <instrlib>:"GENie Meas Output Current.vi"("error"=w392, "VISA"=w393) -> ("error out"=w389:errorcluster, "Output Current"=w391:dbl, "VISA out"=w390:refnum<visa-resource-name>)  [unwired: 7 in]
                        n161 = Wait (ms)(milliseconds to wait=u32 2000) -> ()  [unwired: 1 out]
                        n162 = property on="Seta Carga" class="Bool (strict)"("Value"=TRUE ("Seta Carga")) -> ()  [unwired: 2 in, 2 out]
                        n163 = local write "Corrente de Saída"(w391) -> ()
                      }
                    }
                    n164 = Less Or Equal?(x=w369, y=0.0) -> (x <= y?=w373:bool)
                  }
                }
                frame #1 {
                  n165 = Wait (ms)(milliseconds to wait=u32 1500) -> ()  [unwired: 1 out]
                }
                frame #2 {
                  w400 = FALSE ("Output ON")
                  w403 = refnum<k21> "resfriamento_freio"  # DAQmx Task Name
                  n166 = local write "Liga Fonte"(w400) -> ()
                  n167 = local write "Seta Carga"(w400) -> ()
                  n168 = call <instrlib>:"GENie Config Output On-Off.vi"("error"=w401, "Output ON"=w400, "VISA"=w402) -> ("error out"=w399:errorcluster, "VISA out"=w398:refnum<visa-resource-name>)  [unwired: 7 in]
                  n169 = call-poly <vilib>:"DAQmx Write.vi"("task/channels in"=w403, "data"=w400) -> ()  [unwired: 11 in, 3 out]
                }
              }
            }
            event "Seta Carga": Value Change {
              n170 = event-data() -> ("NewVal"=w408:bool)  [unwired: 1 in, 5 out]
              n171 = local write "Seta Carga"(w408) -> ()
              n172 = local read "Manual?"() -> (w405:bool)
              n173 = case shown="False" w405 {
                tunnel: [0.0 ("Limite Corrente") w415] -> w404
                frame False {
                }
                frame True {
                  n174 = local read "Limite Corrente"() -> (w415:dbl)
                }
              }
              n175 = local read "Limite Tensao"() -> (w413:dbl)
              n176 = call <instrlib>:"GENie Config Current Limit.vi"("error"=w411, "Current Limit"=w404, "VISA"=w412) -> ("error out"=w409:errorcluster, "VISA out"=w410:refnum<visa-resource-name>)  [unwired: 7 in]
              n177 = call <instrlib>:"GENie Config Voltage Limit.vi"("error"=w409, "Volt Limit"=w413, "VISA"=w410) -> ("error out"=w407:errorcluster, "VISA out"=w406:refnum<visa-resource-name>)  [unwired: 7 in]
            }
          }
          n178 = local read "PARAR WHILE"() -> (w345:bool)
        }
      }
    }
    n179 = local read "PARAR WHILE"() -> (w295:bool)
  }
  n180 = while "Aquisição de dados da fonte" {
    shift-right: [w416] -> _
    shift-left: w29 -> [w423]
    tunnel: w27 -> [w424]
    stop <- w417 stop-if-true
    # "Aquisição de dados da fonte"
    n181 = call <instrlib>:"GENie Meas Output Current.vi"("error"=w423, "VISA"=w424) -> ("error out"=w420:errorcluster, "Output Current"=w422:dbl, "VISA out"=w421:refnum<visa-resource-name>)  [unwired: 7 in]
    n182 = Wait (ms)(milliseconds to wait=u32 1500) -> ()  [unwired: 1 out]
    n183 = local write "Corrente de Saída"(w422) -> ()
    n184 = call <instrlib>:"GENie Meas Output Voltage.vi"("error"=w420, "VISA"=w421) -> ("error out"=w416:errorcluster, "Output Voltage"=w419:dbl)  [unwired: 7 in, 1 out]
    n185 = local write "Tensão de Saída"(w419) -> ()
    n186 = local read "PARAR WHILE"() -> (w417:bool)
  }
  n187 = call <vilib>:"DAQmx Start Task.vi"("task/channels in"=w70) -> ("task out"=w41:refnum<k21>)  [unwired: 13 in, 1 out]
  n188 = call <vilib>:"DAQmx Start Task.vi"("task/channels in"=w73) -> ("task out"=w42:refnum<k21>)  [unwired: 13 in, 1 out]
  n189 = call <instrlib>:"Initialize.vi"("VISA resource name"=refnum<visa-resource-name> "GPIB0::1::INSTR") -> ("VISA resource name out"=w49:refnum<visa-resource-name>, "error out"=w48:errorcluster)  [unwired: 13 in]
  n190 = call <vilib>:"DAQmx Start Task.vi"("task/channels in"=w58) -> ("task out"=w57:refnum<k21>)  [unwired: 13 in, 1 out]
  n191 = Initialize Array(FALSE, 4 ("dimension size")) -> (w52:bool[])
  n192 = while {
    tunnel: w57 -> [w428]
    tunnel: [w427] -> w55
    shift-right: [w426] -> _
    shift-left: w52 -> [w429]
    stop <- w425 stop-if-true
    # "Braços de resistores"
    n193 = event shown="[1] \"Resistor 1 MOSFET\": Value Change" {
      selector: _ -> [_ _ _ _ _]
      dyn-events: _ -> [_ _ _ _ _]
      timeout: _ -> [_ _ _ _ _]
      tunnel: w429 -> [_ w435 w440 w446 w452]
      tunnel: w428 -> [_ w432 w438 w444 w450]
      tunnel: [_ w431 w436 w443 w449] -> w427
      tunnel: [_ w430 w437 w442 w448] -> w426
      event Timeout {
        n194 = event-data() -> ()  [unwired: 1 in, 3 out]
      }
      event "Resistor 1 MOSFET": Value Change {
        n195 = event-data() -> ("NewVal"=w433:bool)  [unwired: 1 in, 2 out]
        n196 = Replace Array Subset(array=w435, new element=w433, index=0) -> (w430:bool[])
        n197 = call-poly <vilib>:"DAQmx Write.vi"("task/channels in"=w432, "data"=w430) -> ("task out"=w431:refnum<k21>)  [unwired: 11 in, 2 out]
      }
      event "Resistor 1  047": Value Change {
        n198 = event-data() -> ("NewVal"=w439:bool)  [unwired: 1 in, 2 out]
        n199 = Replace Array Subset(array=w440, new element=w439, index=1) -> (w437:bool[])
        n200 = call-poly <vilib>:"DAQmx Write.vi"("task/channels in"=w438, "data"=w437) -> ("task out"=w436:refnum<k21>)  [unwired: 11 in, 2 out]
      }
      event "Resistor 2 047": Value Change {
        n201 = event-data() -> ("NewVal"=w445:bool)  [unwired: 1 in, 2 out]
        n202 = Replace Array Subset(array=w446, new element=w445, index=2) -> (w442:bool[])
        n203 = call-poly <vilib>:"DAQmx Write.vi"("task/channels in"=w444, "data"=w442) -> ("task out"=w443:refnum<k21>)  [unwired: 11 in, 2 out]
      }
      event "Resistor 2 068": Value Change {
        n204 = event-data() -> ("NewVal"=w451:bool)  [unwired: 1 in, 5 out]
        n205 = Replace Array Subset(array=w452, new element=w451, index=3) -> (w448:bool[])
        n206 = call-poly <vilib>:"DAQmx Write.vi"("task/channels in"=w450, "data"=w448) -> ("task out"=w449:refnum<k21>)  [unwired: 11 in, 2 out]
      }
    }
    n207 = local read "PARAR WHILE"() -> (w425:bool)
  }
  n208 = Initialize Array(FALSE, 7 ("dimension size")) -> (w38:bool[])
  n209 = Initialize Array(TRUE, 7 ("dimension size")) -> (w35:bool[])
  n210 = call-poly <vilib>:"DAQmx Write.vi"("task/channels in"=w41, "data"=w38) -> ("task out"=w44:refnum<k21>)  [unwired: 11 in, 2 out]
  n211 = call-poly <vilib>:"DAQmx Write.vi"("task/channels in"=w42, "data"=w35) -> ("task out"=w43:refnum<k21>)  [unwired: 11 in, 2 out]
  n212 = call <instrlib>:"Config Current.vi"("VISA resource name"=w49, "Element (0: ALL)"=w47, "A Terminal (0: 5A)"=w46, "A Range (7:10)"=w45, "error in (no error)"=w48) -> ("VISA resource name out"=w50:refnum<visa-resource-name>, "error out"=w51:errorcluster)  [unwired: 9 in]
  n213 = while {
    shift-right: [w455] -> _
    shift-left: Enum_Estados_Ensaio."Idle" ("Enum") -> [w472]
    tunnel: w43 -> [w468]
    tunnel: w44 -> [w467]
    tunnel: [w466] -> w67
    tunnel: [w465] -> w66
    shift-right: [w464] -> _
    shift-left: 0.0 -> [w463]
    tunnel: w50 -> [w462]
    tunnel: [w461] -> w61
    shift-right: [w459] -> w63
    shift-left: w51 -> [w460]
    shift-right: [w458] -> _
    shift-left: u32 0 ("millisecond timer value") -> [w457]
    stop <- "PARAR WHILE" stop-if-true
    # "Máquina de estados do ensaio"
    n214 = case shown="\"Ensaio\"" w472 {
      tunnel: [w479 Enum_Estados_Ensaio."Aguarda_PreCarga" ("Enum") w497 Enum_Estados_Ensaio."Delay_PosBracos" ("Enum") w528 Enum_Estados_Ensaio."Aciona_Motor" ("Enum") Enum_Estados_Ensaio."Aguarda_Motor" ("Enum") w563 Enum_Estados_Ensaio."Motor_Rodando" ("Enum") Enum_Estados_Ensaio."Idle" ("Enum") Enum_Estados_Ensaio."Idle" ("Enum") w676] -> w471
      tunnel: w468 -> [w477 w489 w507 w524 w536 w543 w555 w572 w585 w647 w656 w687]
      tunnel: w467 -> [w478 w493 w508 w522 w537 w548 w556 w573 w576 w648 w651 w667]
      tunnel: [w478 w493 w508 w521 w537 w548 w556 w573 w576 w648 w650 w666] -> w465
      tunnel: [w477 w486 w507 w524 w536 w542 w555 w572 w585 w647 w655 w687] -> w466
      tunnel: [w476 w488 w505 w519 w529 w547 w553 w567 w584 w646 w664 w686] -> w464
      tunnel: w463 -> [w476 _ w505 _ w529 w547 _ w567 w584 w646 w664 w686]
      tunnel: w462 -> [w475 w485 w496 w518 w527 w540 w552 w562 w582 w644 w662 w685]
      tunnel: [w475 w485 w496 w518 w527 w540 w552 w562 w578 w644 w662 w685] -> w461
      tunnel: [w474 w484 w495 w517 w526 w539 w551 w561 w579 w643 w661 w684] -> w459
      tunnel: w460 -> [w474 w484 w495 w517 w526 w539 w551 w561 w581 w643 w661 w684]
      tunnel: [w473 w483 w494 w516 w525 w538 w550 w560 w580 w642 w660 w683] -> w458
      tunnel: w457 -> [w473 w483 w494 w516 w525 w538 w550 w560 _ w642 w660 w683]
      tunnel: "Qtd. Braços Ativos" -> [_ _ _ w509 _ _ _ _ _ _ _ w668]
      frame "Idle", Default {
        n215 = Select(t=Enum_Estados_Ensaio."Pre_Carga" ("Enum"), s="Iniciar Acionamento", f=Enum_Estados_Ensaio."Idle" ("Enum")) -> (s? t:f=w479:T4)
      }
      frame "Pre_Carga" {
        n216 = Initialize Array(FALSE, 7 ("dimension size")) -> (w492:bool[])
        n217 = call-poly <vilib>:"DAQmx Write.vi"("task/channels in"=w489, "data"=w492) -> ("task out"=w486:refnum<k21>)  [unwired: 11 in, 2 out]
        n218 = Tick Count (ms)() -> (millisecond timer value=w488:u32)
      }
      frame "Aguarda_PreCarga" {
        n219 = Tick Count (ms)() -> (millisecond timer value=w506:u32)
        n220 = Subtract(x=w506, y=w505) -> (x-y=w502:dbl)
        n221 = Multiply(x="Tempo de Pré-Carga (s)", y=1000.0) -> (x*y=w501:dbl)
        n222 = Greater Or Equal?(x=w502, y=w501) -> (x >= y?=w500:bool)
        n223 = Select(t=Enum_Estados_Ensaio."Ativa_Bracos" ("Enum"), s=w500, f=Enum_Estados_Ensaio."Aguarda_PreCarga" ("Enum")) -> (s? t:f=w497:T4)
      }
      frame "Ativa_Bracos" {
        n224 = Subtract(x=7, y=w509) -> (x-y=w513:dbl)
        n225 = Initialize Array(TRUE, w509) -> (w512:bool[])
        n226 = Initialize Array(FALSE, w513) -> (w511:bool[])
        n227 = Build Array (concatenate)(w512, w511) -> (w510:bool[])
        n228 = call-poly <vilib>:"DAQmx Write.vi"("task/channels in"=w522, "data"=w510) -> ("task out"=w521:refnum<k21>)  [unwired: 11 in, 2 out]
        n229 = Tick Count (ms)() -> (millisecond timer value=w519:u32)
      }
      frame "Delay_PosBracos" {
        n230 = Tick Count (ms)() -> (millisecond timer value=w535:u32)
        n231 = Subtract(x=w535, y=w529) -> (x-y=w534:dbl)
        n232 = Greater Or Equal?(x=w534, y=1000.0) -> (x >= y?=w533:bool)
        n233 = Select(t=Enum_Estados_Ensaio."Desativa_PreCarga" ("Enum"), s=w533, f=Enum_Estados_Ensaio."Delay_PosBracos" ("Enum")) -> (s? t:f=w528:T4)
      }
      frame "Desativa_PreCarga" {
        n234 = Initialize Array(TRUE, 7 ("dimension size")) -> (w546:bool[])
        n235 = call-poly <vilib>:"DAQmx Write.vi"("task/channels in"=w543, "data"=w546) -> ("task out"=w542:refnum<k21>)  [unwired: 11 in, 2 out]
      }
      frame "Aciona_Motor" {
        n236 = local write "velocidade"(u16 3500 ("velocidade")) -> ()
        n237 = Tick Count (ms)() -> (millisecond timer value=w553:u32)
      }
      frame "Aguarda_Motor" {
        n238 = Tick Count (ms)() -> (millisecond timer value=w571:u32)
        n239 = Subtract(x=w571, y=w567) -> (x-y=w558:dbl)
        n240 = Divide(x=w558, y=1000.0) -> (x/y=→"Tempo Decorrido Acionamento Motor":dbl)
        n241 = Multiply(x="Tempo de Acionamento do Motor (s)", y=1000.0) -> (x*y=w564:dbl)
        n242 = Greater Or Equal?(x=w558, y=w564) -> (x >= y?=w570:bool)
        n243 = Select(t=Enum_Estados_Ensaio."Motor_Rodando" ("Enum"), s=w570, f=Enum_Estados_Ensaio."Aguarda_Motor" ("Enum")) -> (s? t:f=w563:T4)
      }
      frame "Ensaio" {
        n244 = flat-sequence {
          tunnel: w582 -> [w588]
          tunnel: w581 -> [w587]
          tunnel: [w590] -> w580
          tunnel: [w589] -> w577
          tunnel: [w586] -> w575
          tunnel: [w594] -> w579
          tunnel: [w595] -> w578
          tunnel: w577 -> [w596]
          tunnel: w575 -> [w591]
          frame #0 {
            n245 = call <instrlib>:"Wait Update.vi"("VISA resource name"=w588, "error in (no error)"=w587) -> ("VISA resource name out"=w589:refnum<visa-resource-name>, "error out"=w586:errorcluster)  [unwired: 12 in]
            n246 = Tick Count (ms)() -> (millisecond timer value=w590:u32)
          }
          frame #1 {
            n247 = Tick Count (ms)() -> (millisecond timer value=w607:u32)
            n248 = while {
              tunnel: w596 -> [w640]
              shift-right: [w626] -> w604
              shift-left: w591 -> [w639]
              tunnel: w607 -> [w632]
              tunnel: [w627] -> w605
              stop <- w628 stop-if-true
              n249 = call <instrlib>:"Query Condition Status.vi"("VISA resource name"=w640, "error in (no error)"=w639) -> ("VISA resource name out"=w627:refnum<visa-resource-name>, "Condition"=w638:i32, "error out"=w626:errorcluster)  [unwired: 11 in]
              n250 = Tick Count (ms)() -> (millisecond timer value=w633:u32)
              n251 = Subtract(x=w633, y=w632) -> (x-y=w631:u32)
              n252 = And(x=w638, y=1) -> (x .and. y?=w635:i32)
              n253 = local read "ABORTAR"() -> (w624:bool)
              n254 = Equal?(x=w635, y=0) -> (x = y?=w634:bool)
              n255 = Greater Or Equal?(x=w631, y=u32 30000) -> (x >= y?=w625:bool)
              n256 = Or(x=w634, y=w624) -> (x .or. y?=w629:bool)
              n257 = Or(x=w629, y=w625) -> (x .or. y?=w628:bool)
            }
            n258 = for {
              N: 6 -> [_]
              tunnel: w605 -> [w622]
              shift-right: [w613] -> w594
              shift-left: w604 -> [w623]
              tunnel: [w612] -> w603 mode=indexing
              tunnel: [w611] -> w595
              i -> [w617]
              w618 = u32 100000 ("End Point (1000)")
              w619 = u32 0 ("Start Point (0)")
              n259 = Increment(x=w617) -> (x+1=w616:i32)
              n260 = call <instrlib>:"Config Waveform.vi"("VISA resource name"=w622, "End Point (1000)"=w618, "Start Point (0)"=w619, "Select Trace (1)"=w616, "error in (no error)"=w623) -> ("VISA resource name out"=w621:refnum<visa-resource-name>, "error out"=w620:errorcluster)  [unwired: 9 in]
              n261 = call <instrlib>:"Read Range.vi"("VISA resource name"=w621, "error in (no error)"=w620) -> ("VISA resource name out"=w611:refnum<visa-resource-name>, "Range"=w614:dbl, "error out"=w613:errorcluster)  [unwired: 11 in]
              n262 = call <instrlib>:"Read Waveform.vi"("VISA resource name"=w611, "End Point (1000)"=w618, "Start Point (0)"=w619, "Select Trace (1)"=w616, "error in (no error)"=w613) -> ("Waveform Data"=w615:string)  [unwired: 8 in, 2 out]
              n263 = call <instrlib>:"Waveform Data Convert.vi"("Input Data"=w615, "Range"=w614) -> ("Output"=w612:dbl[])  [unwired: 11 in, 2 out]
            }
            n264 = call "waveform_demux.vi"("Output"=w603) -> ("Corrente"=w592:dbl[][], "Tensão"=w593:dbl[][])  [unwired: 9 in]
            "Corrente" <- w592
            "Tensão" <- w593
            n265 = Transpose 2D Array(2D array=w593) -> (transposed array=w597:dbl[][])
            n266 = Transpose 2D Array(2D array=w592) -> (transposed array=w598:dbl[][])
            n267 = for {
              tunnel: w597 -> [w610] mode=indexing
              tunnel: w598 -> [w609] mode=indexing
              tunnel: [w608] -> w599 mode=indexing
              n268 = Build Array (concatenate)(w610, w609) -> (w608:dbl[])
            }
            n269 = call-poly <vilib>:"Write Delimited Spreadsheet.vi"("file path (dialog if empty)"="Salvar Ensaio", "format (%.3f)"="%.3f", "2D data"=w599, "delimiter (\\t)"=";" ("delimiter (\\t)")) -> ()  [unwired: 10 in, 2 out]
          }
        }
        n270 = local write "Ensaio Rodando"(TRUE ("Ensaio Rodando")) -> ()
      }
      frame "Para_Motor" {
        n271 = local write "velocidade"(u16 0 ("velocidade")) -> ()
      }
      frame "Emergencia\n" {
        n272 = Initialize Array(FALSE, 7 ("dimension size")) -> (w654:bool[])
        n273 = Initialize Array(TRUE, 7 ("dimension size")) -> (w659:bool[])
        n274 = local write "velocidade"(u16 0 ("velocidade")) -> ()
        n275 = call-poly <vilib>:"DAQmx Write.vi"("task/channels in"=w651, "data"=w654) -> ("task out"=w650:refnum<k21>)  [unwired: 11 in, 2 out]
        n276 = call-poly <vilib>:"DAQmx Write.vi"("task/channels in"=w656, "data"=w659) -> ("task out"=w655:refnum<k21>)  [unwired: 11 in, 2 out]
      }
      frame "Motor_Rodando" {
        n277 = Subtract(x=7, y=w668) -> (x-y=w672:dbl)
        n278 = Initialize Array(TRUE, w668) -> (w671:bool[])
        n279 = Initialize Array(FALSE, w672) -> (w670:bool[])
        n280 = Build Array (concatenate)(w671, w670) -> (w669:bool[])
        n281 = call-poly <vilib>:"DAQmx Write.vi"("task/channels in"=w667, "data"=w669) -> ("task out"=w666:refnum<k21>)  [unwired: 11 in, 2 out]
        n282 = local write "Ensaio Rodando"(FALSE ("Ensaio Rodando")) -> ()
        n283 = Select(t=Enum_Estados_Ensaio."Ensaio" ("Enum"), s="Iniciar Ensaio", f=Enum_Estados_Ensaio."Motor_Rodando" ("Enum")) -> (s? t:f=w679:T4)
        n284 = Select(t=Enum_Estados_Ensaio."Para_Motor" ("Enum"), s="Finalizar Sessão", f=w679) -> (s? t:f=w676:T4)
      }
    }
    n285 = Select(t=Enum_Estados_Ensaio."Emergencia\n" ("Enum"), s="ABORTAR", f=w471) -> (s? t:f=w455:T4)
    "Estado Atual" <- w455
  }
  n286 = call <vilib>:"DAQmx Stop Task.vi"("task/channels in"=w55) -> ("task out"=w56:refnum<k21>)  [unwired: 13 in, 1 out]
  n287 = call <vilib>:"DAQmx Clear Task.vi"("task in"=w56) -> ()  [unwired: 14 in, 1 out]
  n288 = call-dynamic "Close Session.vi"("MB_Serial session"=w21) -> ()  [unwired: 10 in, 1 out]
  n289 = call <instrlib>:"Close.vi"("VISA resource name"=w61, "error in (no error)"=w63) -> ()  [unwired: 13 in, 1 out]
  n290 = call <vilib>:"DAQmx Stop Task.vi"("task/channels in"=w66) -> ("task out"=w68:refnum<k21>)  [unwired: 13 in, 1 out]
  n291 = call <vilib>:"DAQmx Stop Task.vi"("task/channels in"=w67) -> ("task out"=w69:refnum<k21>)  [unwired: 13 in, 1 out]
  n292 = call <vilib>:"DAQmx Clear Task.vi"("task in"=w68) -> ()  [unwired: 14 in, 1 out]
  n293 = call <vilib>:"DAQmx Clear Task.vi"("task in"=w69) -> ()  [unwired: 14 in, 1 out]
  n294 = call <instrlib>:"GENie Close.vi"("error"=w28, "VISA name"=w31) -> ()  [unwired: 9 in, 1 out]
